vi "Waveform Set.vi"(6 "Update":bool=TRUE, 7 "Function":u8=1, 8 "error in (no error)":errorcluster, 9 "node":i32, 10 "idxChannel":i32, 11 "hdwf":i32) -> (0 "error out":errorcluster, 1 "func_out":i32)   [LabVIEW 2024, in "AD2 DLL.lvlib"]
uses:
  AD2 DLL.lvlib
  <vilib>/Digilent/AD2 Toolkit/AD2.lvlib
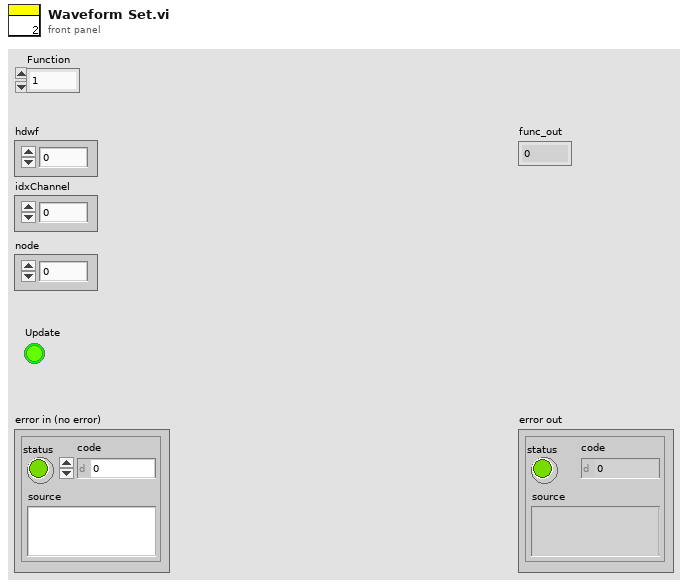
[diagram p1: front panel]
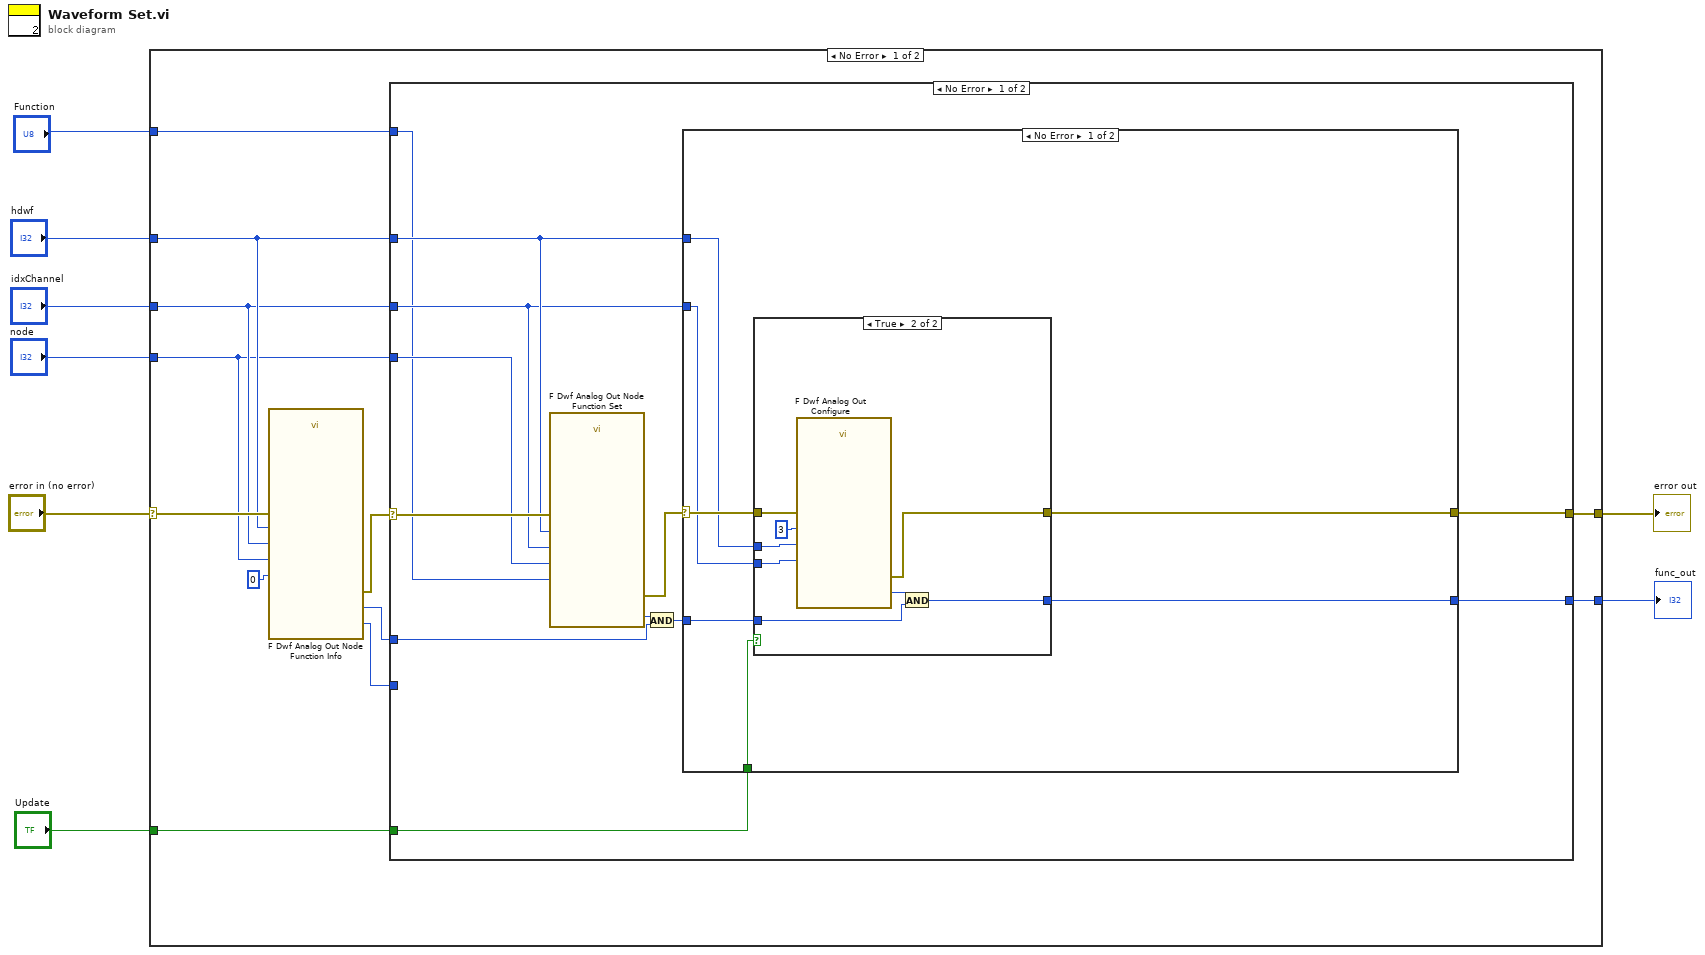
[diagram p0: block diagram]
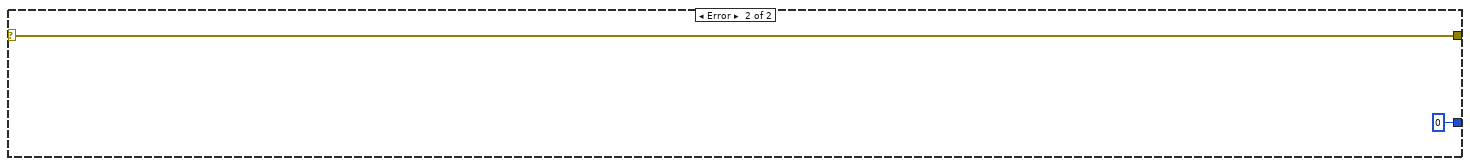
[diagram p5: hidden frame]
diagram:
  n1 = case shown="No Error" "error in (no error)" {
    selector: "error in (no error)" -> [w15 w55]
    tunnel: [w19 w55] -> w8
    tunnel: "hdwf" -> [w13 _]
    tunnel: "idxChannel" -> [w12 _]
    tunnel: "node" -> [w11 _]
    tunnel: "Function" -> [w20 _]
    tunnel: [w18 0] -> w3
    tunnel: "Update" -> [w17 _]
    frame No Error {
      n2 = call <vilib>:"F Dwf Analog Out Node Function Info.vi"("pfsfunc"=0, "error in (no error)"=w15, "node"=w11, "idxChannel"=w12, "hdwf"=w13) -> ("error out"=w14:errorcluster, "function return"=w16:i32, "pfsfunc out"=w9:i32)  [unwired: 4 in]
      n3 = case shown="No Error" w14 {
        selector: w14 -> [w25 w53]
        tunnel: w20 -> [w21 _]
        tunnel: [w32 w53] -> w19
        tunnel: w13 -> [w24 _]
        tunnel: w12 -> [w23 _]
        tunnel: w11 -> [w22 _]
        tunnel: w16 -> [w31 w52]
        tunnel: [w29 w52] -> w18
        tunnel: w17 -> [w28 _]
        tunnel: w9 -> [_ _]
        frame No Error {
          n4 = call <vilib>:"F Dwf Analog Out Node Function Set.vi"("func"=w21, "error in (no error)"=w25, "node"=w22, "idxChannel"=w23, "hdwf"=w24) -> ("error out"=w27:errorcluster, "function return"=w26:i32)  [unwired: 5 in]
          n5 = And(x=w26, y=w31) -> (x .and. y?=w30:i32)
          n6 = case shown="No Error" w27 {
            selector: w27 -> [w39 w51]
            tunnel: [w36 w51] -> w32
            tunnel: w24 -> [w38 _]
            tunnel: w23 -> [w37 _]
            tunnel: w30 -> [w35 w50]
            tunnel: [w34 w50] -> w29
            tunnel: w28 -> [w33 _]
            frame No Error {
              n7 = case shown="True" w33 {
                tunnel: w39 -> [w41 w49]
                tunnel: w38 -> [_ w47]
                tunnel: w37 -> [_ w46]
                tunnel: [w41 w45] -> w36
                tunnel: w35 -> [w40 w43]
                tunnel: [w40 w42] -> w34
                frame False {
                }
                frame True {
                  n8 = call <vilib>:"F Dwf Analog Out Configure.vi"("error in (no error)"=w49, "fStart"=3, "idxChannel"=w46, "hdwf"=w47) -> ("error out"=w45:errorcluster, "function return"=w44:i32)  [unwired: 6 in]
                  n9 = And(x=w44, y=w43) -> (x .and. y?=w42:i32)
                }
              }
            }
            frame Error {
            }
          }
        }
        frame Error {
        }
      }
    }
    frame Error {
    }
  }
  "error out" <- w8
  "func_out" <- w3
